vi "DB and WB to RH.vi"(1 "Wet Bulb Temp [DegF]":dbl, 2 "Dry Bulb Temp [DegF]":dbl) -> (0 "Relative Humidity [-]":dbl)   [LabVIEW 2020]
panel:
  out "ew":dbl
  out "ed":dbl
  # "http://www.1728.org/relhum.htm"
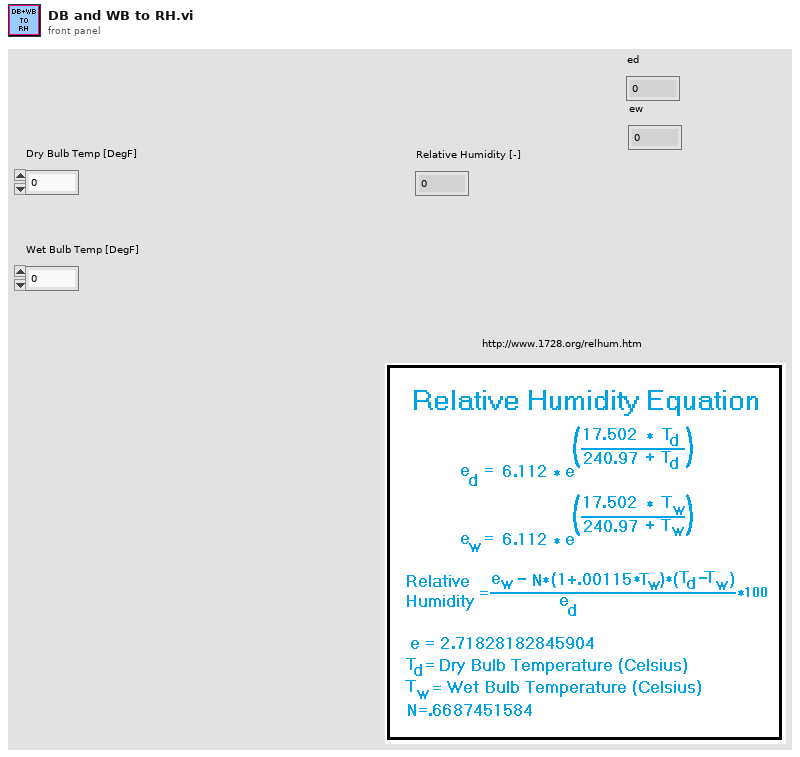
[diagram p1: front panel]
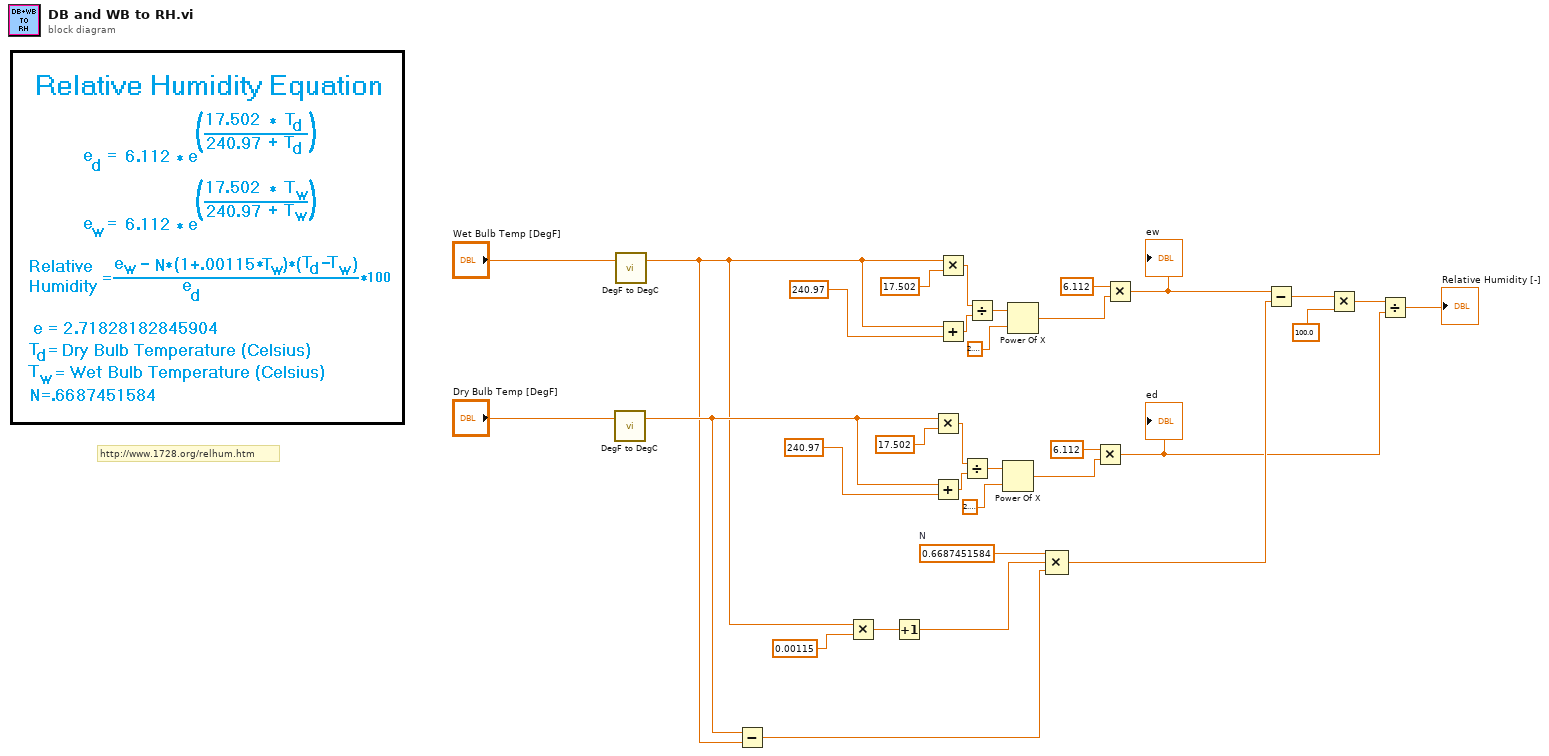
[diagram p0: block diagram]
diagram:
  w16 = 0.6687451584  # N
  # "http://www.1728.org/relhum.htm"
  n1 = call "DegF to DegC.vi"("Input Temperature in Fahrenheit"="Dry Bulb Temp [DegF]") -> ("Output Temperature in Celcius"=w11:dbl)  [unwired: 1 in, 1 out]
  n2 = call "DegF to DegC.vi"("Input Temperature in Fahrenheit"="Wet Bulb Temp [DegF]") -> ("Output Temperature in Celcius"=w9:dbl)  [unwired: 1 in, 1 out]
  n3 = Subtract(x=w11, y=w9) -> (x-y=w7:dbl)
  n4 = Multiply(x=w9, y=0.00115) -> (x*y=w15:dbl)
  n5 = Increment(x=w15) -> (x+1=w13:dbl)
  n6 = Multiply(x=w11, y=17.502) -> (x*y=w29:dbl)
  n7 = Add(x=w11, y=240.97) -> (x+y=w28:dbl)
  n8 = Multiply(x=w9, y=17.502) -> (x*y=w20:dbl)
  n9 = Add(x=w9, y=240.97) -> (x+y=w21:dbl)
  n10 = Divide(x=w29, y=w28) -> (x/y=w26:dbl)
  n11 = Divide(x=w20, y=w21) -> (x/y=w23:dbl)
  n12 = Power Of X(1:2.718281828459045, 2:w26) -> (0:w18:dbl)
  n13 = Power Of X(1:2.718281828459045, 2:w23) -> (0:w17:dbl)
  n14 = Compound Arithmetic op=MULTIPLY(w16, w13, w7) -> (w6:dbl)
  n15 = Multiply(x=6.112, y=w18) -> (x*y=w2:dbl)
  "ed" <- w2
  n16 = Multiply(x=6.112, y=w17) -> (x*y=w8:dbl)
  "ew" <- w8
  n17 = Subtract(x=w8, y=w6) -> (x-y=w5:dbl)
  n18 = Multiply(x=w5, y=100.0) -> (x*y=w3:dbl)
  n19 = Divide(x=w3, y=w2) -> (x/y=→"Relative Humidity [-]":dbl)
